vi "Corrente.vi"() -> ()   [LabVIEW 2025]
panel:
  out "Error out Fonte 3":errorcluster
  in  "?":enum32{"Controle", "Error out"}(tab)
  in  "Endereço Agilent 6680A":i16
  in  "?":bool
  in  "Corrente Inicial":dbl format="%#_6p"
  in  "Acréscimo":dbl format="%#_6f"
  in  "Corrente Final":dbl
  in  "Tensão (V)":string
  in  "Ton (ms)":dbl
  in  "Toff (ms)":dbl
  out "Error out Fonte 2":errorcluster
  out "Error out Fonte":errorcluster
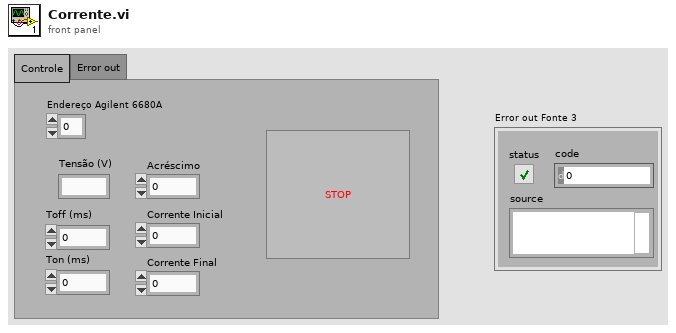
[diagram p1: front panel]
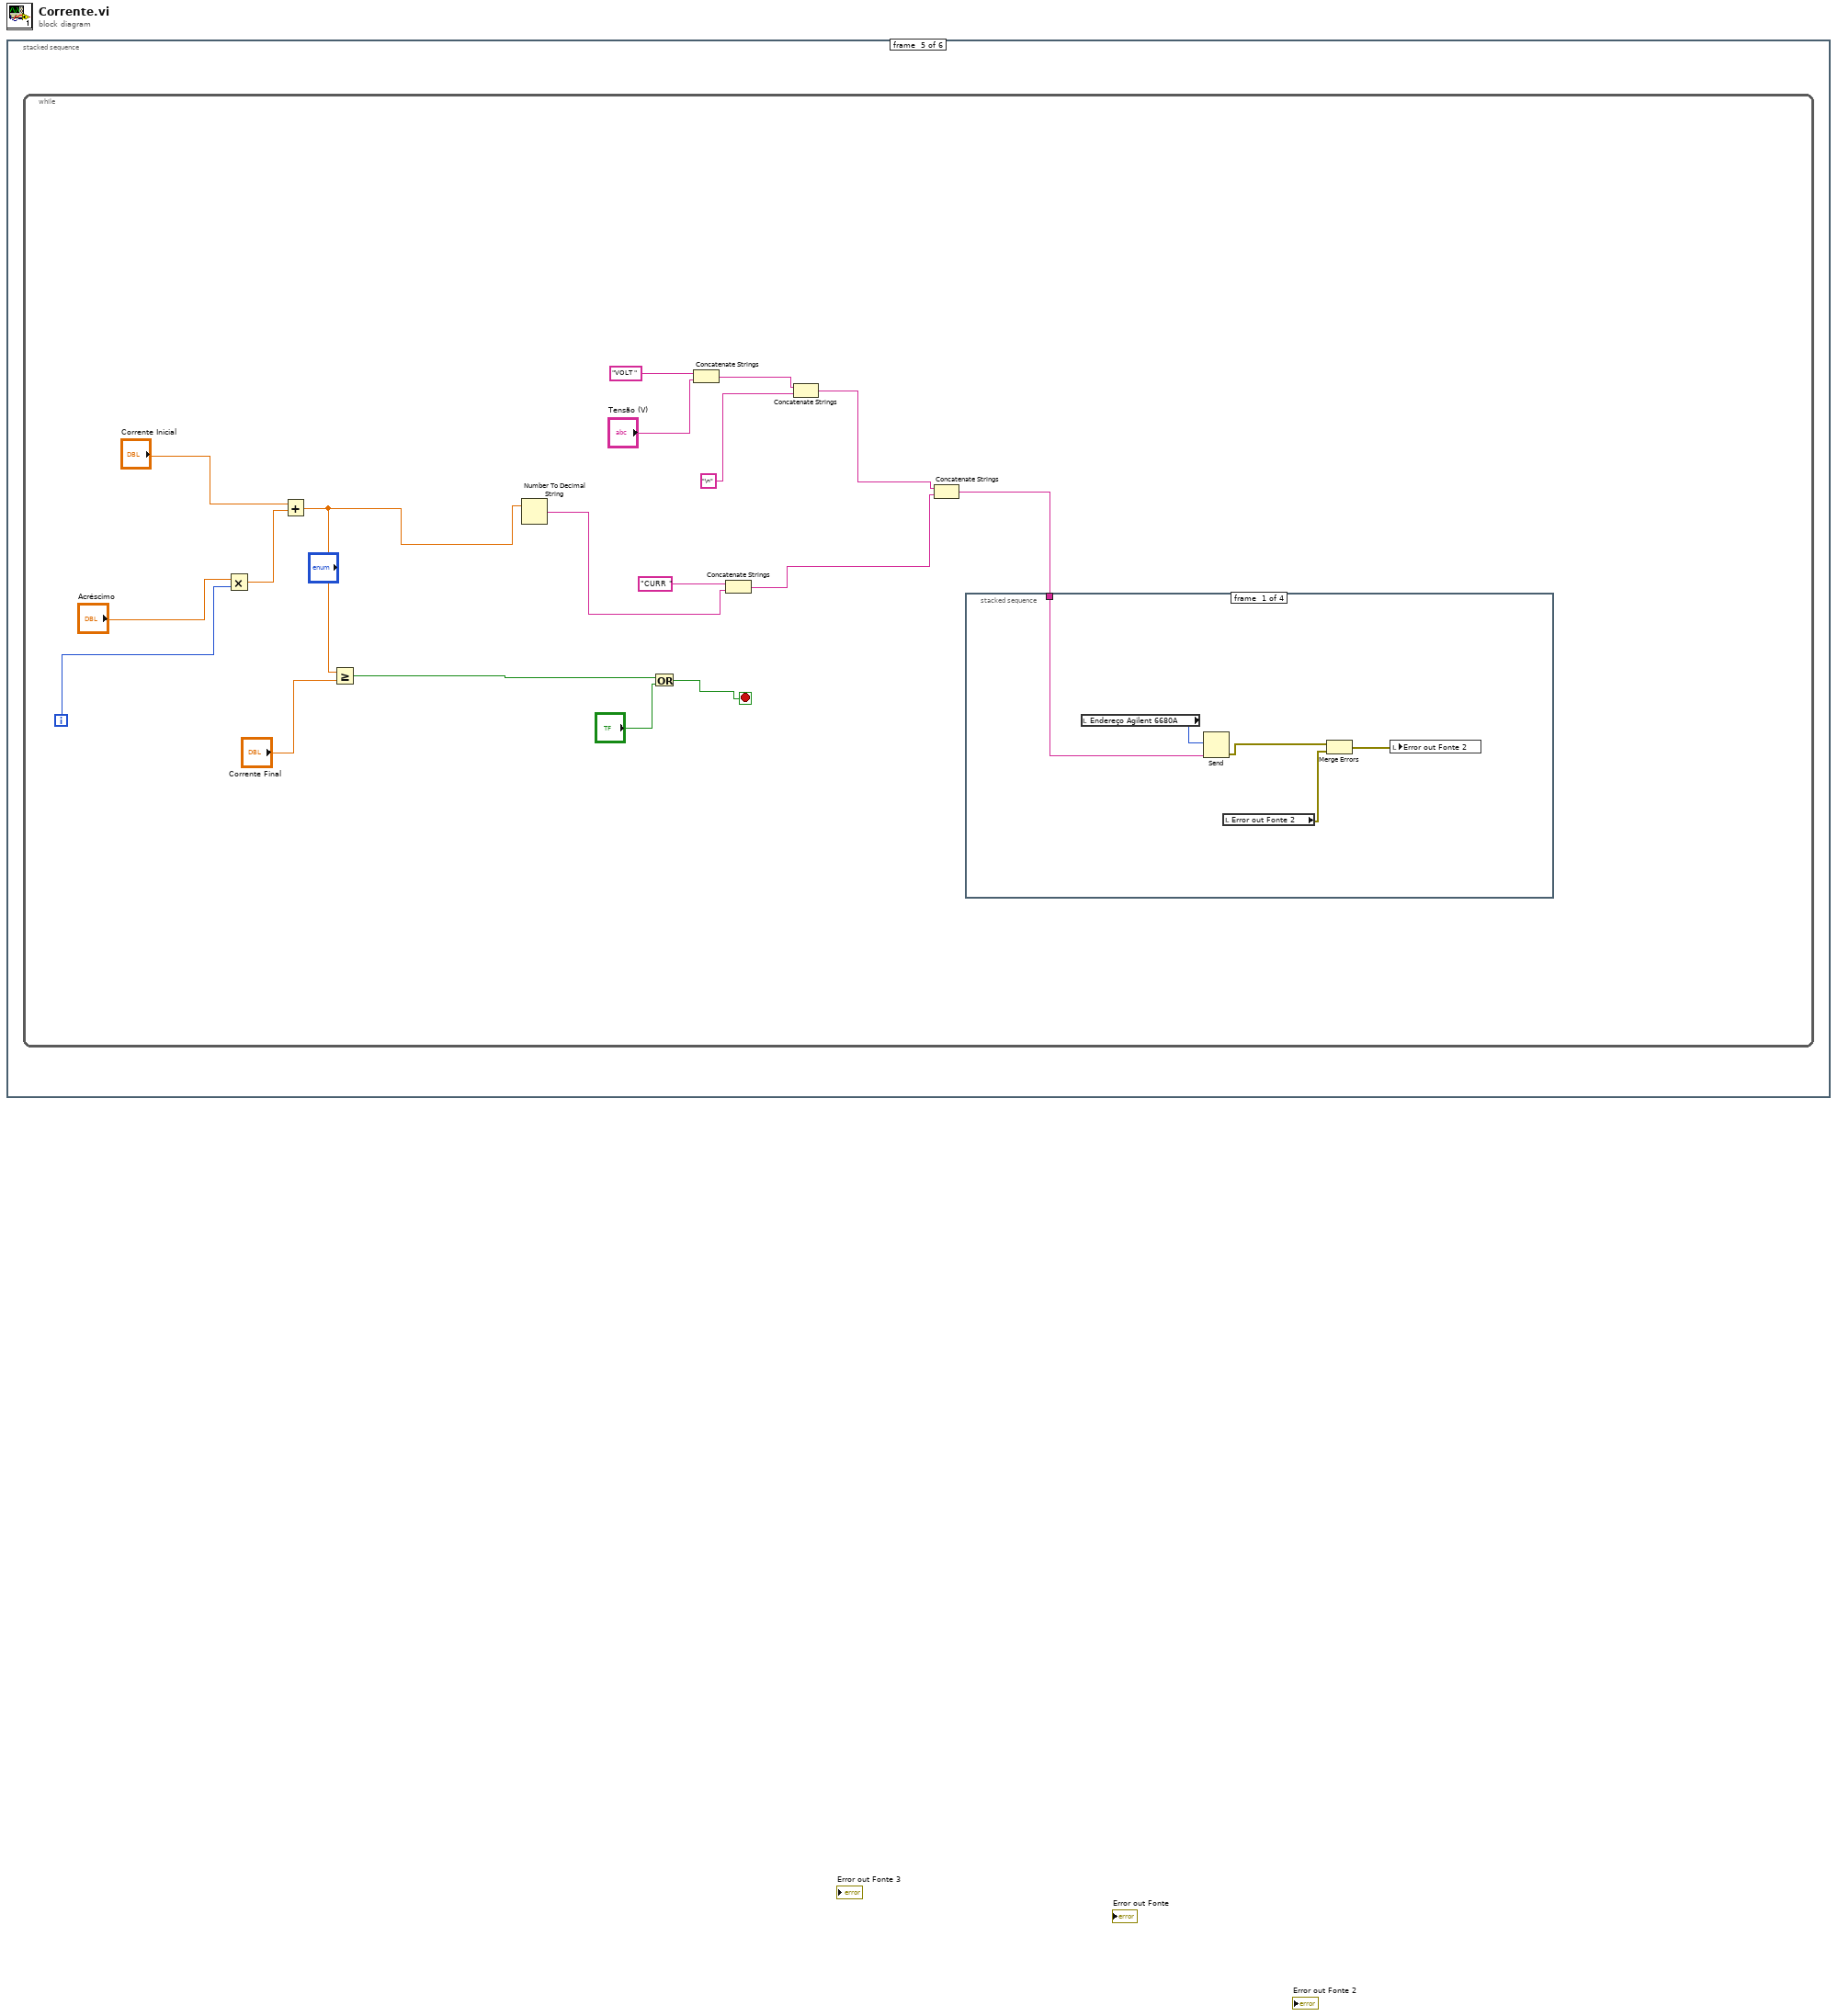
[diagram p0: block diagram]
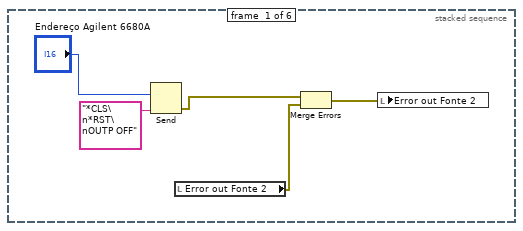
[diagram p2: hidden frame]
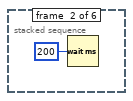
[diagram p3: hidden frame]
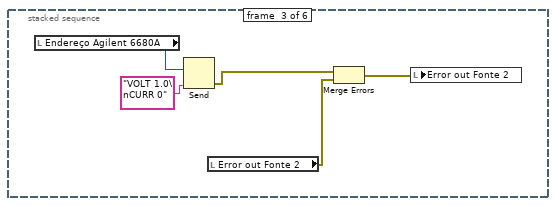
[diagram p4: hidden frame]
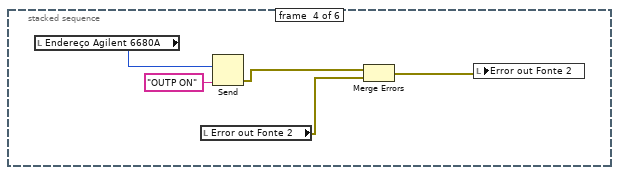
[diagram p5: hidden frame]
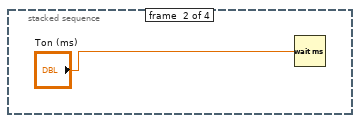
[diagram p6: hidden frame]
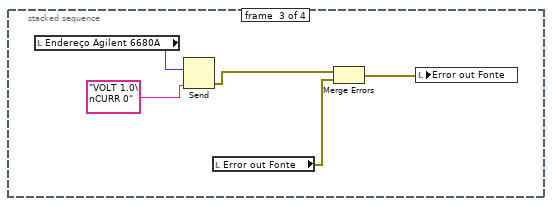
[diagram p7: hidden frame]
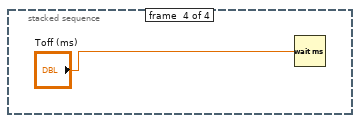
[diagram p8: hidden frame]
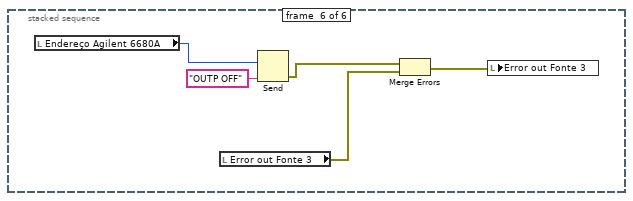
[diagram p9: hidden frame]
diagram:
  n1 = stacked-sequence {
    frame #0 {
      n2 = Send(2:"Endereço Agilent 6680A", 5:"*CLS\n*RST\nOUTP OFF" ("data string")) -> (8:w5:errorcluster)  [unwired: 3 in, 2 out]
      n3 = local read "Error out Fonte 2"() -> (w4:errorcluster)
      n4 = Merge Errors(w5, w4) -> (w1:errorcluster)
      n5 = local write "Error out Fonte 2"(w1) -> ()
    }
    frame #1 {
      n6 = Wait (ms)(milliseconds to wait=u32 200) -> ()  [unwired: 1 out]
    }
    frame #2 {
      n7 = local read "Endereço Agilent 6680A"() -> (w8:i16)
      n8 = Send(2:w8, 5:"VOLT 1.0\nCURR 0" ("data string")) -> (8:w10:errorcluster)  [unwired: 3 in, 2 out]
      n9 = local read "Error out Fonte 2"() -> (w11:errorcluster)
      n10 = Merge Errors(w10, w11) -> (w9:errorcluster)
      n11 = local write "Error out Fonte 2"(w9) -> ()
    }
    frame #3 {
      n12 = local read "Endereço Agilent 6680A"() -> (w12:i16)
      n13 = local read "Error out Fonte 2"() -> (w15:errorcluster)
      n14 = Send(2:w12, 5:"OUTP ON" ("data string")) -> (8:w14:errorcluster)  [unwired: 3 in, 2 out]
      n15 = Merge Errors(w14, w15) -> (w13:errorcluster)
      n16 = local write "Error out Fonte 2"(w13) -> ()
    }
    frame #4 {
      n17 = while {
        i -> [w26]
        stop <- w24 stop-if-true
        n18 = Multiply(x="Acréscimo", y=w26) -> (x*y=w31:dbl)
        n19 = Add(x="Corrente Inicial", y=w31) -> (x+y=w34:dbl)
        n20 = Greater Or Equal?(x=w34, y="Corrente Final") -> (x >= y?=w33:bool)
        n21 = Number To Decimal String(number=w34) -> (decimal integer string=w22:string)  [unwired: 1 in]
        n22 = Or(x=w33, y="?") -> (x .or. y?=w24:bool)
        n23 = Concatenate Strings("VOLT " ("data string"), "Tensão (V)") -> (w20:string)
        n24 = Concatenate Strings("CURR " ("data string"), w22) -> (w18:string)
        n25 = Concatenate Strings(w20, "\n") -> (w19:string)
        n26 = Concatenate Strings(w19, w18) -> (w17:string)
        n27 = stacked-sequence {
          tunnel: w17 -> [w35 _ _ _]
          frame #0 {
            n28 = local read "Endereço Agilent 6680A"() -> (w39:i16)
            n29 = Send(2:w39, 5:w35) -> (8:w37:errorcluster)  [unwired: 3 in, 2 out]
            n30 = local read "Error out Fonte 2"() -> (w36:errorcluster)
            n31 = Merge Errors(w37, w36) -> (w38:errorcluster)
            n32 = local write "Error out Fonte 2"(w38) -> ()
          }
          frame #1 {
            n33 = Wait (ms)(milliseconds to wait="Ton (ms)") -> ()  [unwired: 1 out]
          }
          frame #2 {
            n34 = local read "Endereço Agilent 6680A"() -> (w45:i16)
            n35 = Send(2:w45, 5:"VOLT 1.0\nCURR 0" ("data string")) -> (8:w43:errorcluster)  [unwired: 3 in, 2 out]
            n36 = local read "Error out Fonte"() -> (w42:errorcluster)
            n37 = Merge Errors(w43, w42) -> (w44:errorcluster)
            n38 = local write "Error out Fonte"(w44) -> ()
          }
          frame #3 {
            n39 = Wait (ms)(milliseconds to wait="Toff (ms)") -> ()  [unwired: 1 out]
          }
        }
      }
    }
    frame #5 {
      n40 = local read "Endereço Agilent 6680A"() -> (w48:i16)
      n41 = local read "Error out Fonte 3"() -> (w49:errorcluster)
      n42 = Send(2:w48, 5:"OUTP OFF" ("data string")) -> (8:w50:errorcluster)  [unwired: 3 in, 2 out]
      n43 = Merge Errors(w50, w49) -> (w51:errorcluster)
      n44 = local write "Error out Fonte 3"(w51) -> ()
    }
  }
